vi "getGain.vi"(6 "Delay between send and receive [ms]":i32=100, 8 "error in (no error)":errorcluster, 11 "CCD in":refnum<class "CCD.lvclass">) -> (0 "error out":errorcluster, 1 "gain token":i32, 2 "gain info":string, 3 "CCD out":refnum<class "CCD.lvclass">)   [LabVIEW 2023, in "CCD.lvclass"]
uses:
  CCD.lvclass
  Gain.ctl
  20f7d3bd-08ac-4524-9bed-df36c1da25a0.vi
  a21955fc-e3a0-4e36-8495-41f1bfac7860.vi
  <vilib>/JDP Science/JSONtext/Variant to JSON Text.vi
  <vilib>/JDP Science/JSONtext/Set Item.vi
  <vilib>/JDP Science/JSONtext/JSON text to Variant.vi
  <vilib>/JDP Science/JSONtext/LVClass Serializer/JSONtext LVClass Serializer.lvclass
  CCD.lvclass/CCD.ctl
  GenericDevice/GenericDevice.lvclass
  <vilib>/IlluminatedG/lv-web-crypto/lv-json/JSON/JSON.lvlib
panel:
  # "Connector Pane"
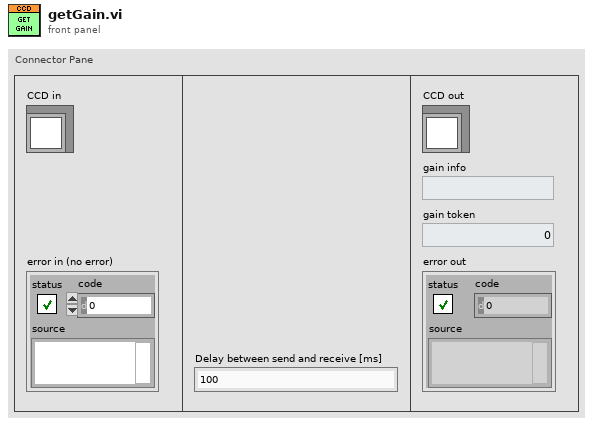
[diagram p1: front panel]
types:
  T1 = typedef "CCD.lvclass/Gain.ctl" = cluster{"info":string, "token":i32}
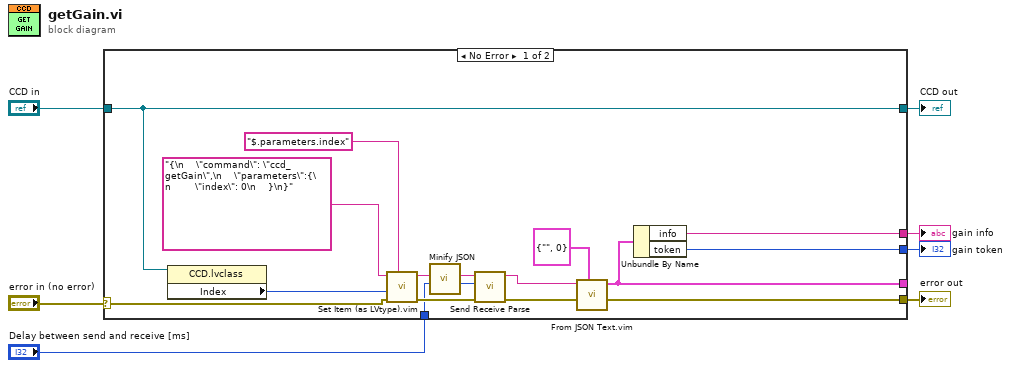
[diagram p0: block diagram]
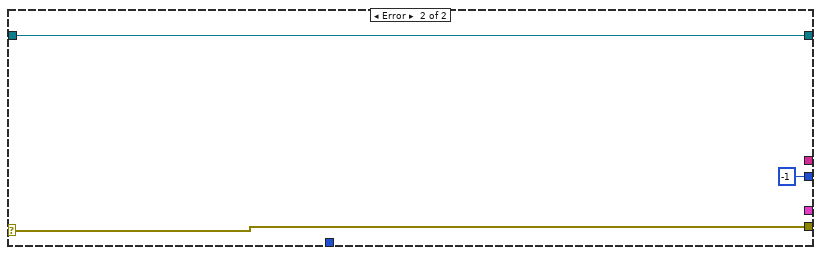
[diagram p2: hidden frame]
diagram:
  n1 = case shown="No Error" "error in (no error)" {
    selector: "error in (no error)" -> [w19 w26]
    tunnel: [w18 w26] -> w6
    tunnel: [w21 w25] -> w4
    tunnel: "CCD in" -> [w21 w25]
    tunnel: [w14 _] -> _
    tunnel: [w13 _] -> w3
    tunnel: [w9 -1 ("token")] -> w1
    tunnel: "Delay between send and receive [ms]" -> [w10 _]
    frame No Error {
      n2 = property class="CCD.lvclass"(reference=w21) -> ("Index"=w20:i32)  [unwired: 1 in, 2 out]
      n3 = call "Set Item (as LVtype).vim"("$Path or Item Name"="$.parameters.index", "error in (no error)"=w19, "Anything"=w20, "JSON"="{\n    \"command\": \"ccd_getGain\",\n    \"parameters\":{\n        \"index\": 0\n    }\n}") -> ("error out"=w15:errorcluster, "<JSON>"=w12:string)  [unwired: 4 in, 1 out]
      n4 = call <vilib>:"Minify JSON.vi"("JSON String"=w12) -> ("Minified JSON"=w11:string)  [unwired: 10 in]
      n5 = call "Send Receive Parse.vi"("error in"=w15, "Delay between send and receive [ms]"=w10, "<JSON>"=w11) -> ("error out"=w16:errorcluster, "results-JSON string"=w17:string)  [unwired: 6 in, 1 out]
      n6 = call "From JSON Text.vim"("Data Type and Default Value"=T1 {"info"="", "token"=0} ("gains"), "error in (no error)"=w16, "JSON"=w17) -> ("error out"=w18:errorcluster, "Data out"=w14:T1)  [unwired: 7 in]
      n7 = Unbundle By Name(w14) -> ("info"=w13:string, "token"=w9:i32)
    }
    frame Error {
    }
  }
  "error out" <- w6
  "CCD out" <- w4
  "gain info" <- w3
  "gain token" <- w1
